vi "Set Operational Mode.vi"(7 "Box ID":u8, 8 "error in (no error)":errorcluster, 9 "Precision Mode":bool, 10 "PID Disable":bool, 11 "CAN in":refnum<class "XNET_BS120x.lvclass">) -> (0 "error out":errorcluster, 3 "CAN out":refnum<class "XNET_BS120x.lvclass">)   [LabVIEW 2021, in "BS120x Driver.lvlib" / "XNET_BS120x.lvclass"]
uses:
  XNET_BS120x.lvclass
  BS120x.lvclass
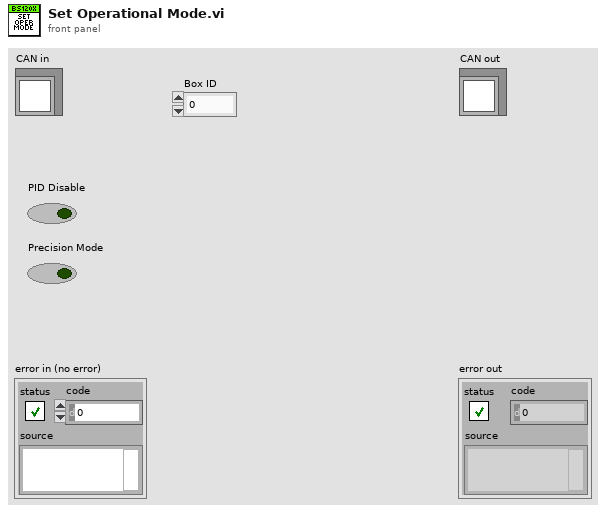
[diagram p1: front panel]
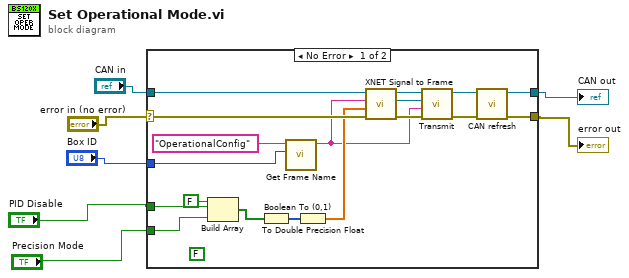
[diagram p0: block diagram]
diagram:
  n1 = case shown="No Error" "error in (no error)" {
    selector: "error in (no error)" -> [w24 w27]
    tunnel: [w18 w27] -> w6
    tunnel: [w16 w26] -> w7
    tunnel: "CAN in" -> [w23 w26]
    tunnel: "Precision Mode" -> [w11 _]
    tunnel: "PID Disable" -> [w10 _]
    tunnel: "Box ID" -> [w14 _]
    frame No Error {
      (unwired) FALSE ("element")
      n2 = Build Array(FALSE ("element"), w10, w11) -> (w9:bool[])
      n3 = Boolean To (0,1)(Boolean=w9) -> (0, 1=w25:i16[])
      n4 = call "Get Frame Name.vi"("Box ID"=w14, "Frame Name"="OperationalConfig" ("name")) -> ("Frame Name out"=w12:string)  [unwired: 9 in]
      n5 = To Double Precision Float(number=w25) -> (double precision float=w13:dbl[])
      n6 = call "XNET Signal to Frame.vi"("error in (no error)"=w24, "Data Array"=w13, "Frame"=w12, "CAN in"=w23) -> ("error out"=w22:errorcluster, "Data"=w21:refnum<class "XNET Data.lvclass">, "CAN out"=w20:refnum<class "XNET_BS120x.lvclass">)  [unwired: 5 in]
      n7 = call "Transmit.vi"("error in (no error)"=w22, "Frame"=w12, "Data in"=w21, "CAN in"=w20) -> ("error out"=w19:errorcluster, "CAN out"=w17:refnum<class "XNET_BS120x.lvclass">)  [unwired: 6 in]
      n8 = call "CAN refresh.vi"("error in (no error)"=w19, "CAN in"=w17) -> ("error out"=w18:errorcluster, "CAN out"=w16:refnum<class "XNET_BS120x.lvclass">)  [unwired: 8 in]
    }
    frame Error {
    }
  }
  "error out" <- w6
  "CAN out" <- w7
